vi "gauge_panel.vi"() -> ()   [LabVIEW 2017]
uses:
  slide_indicator.ctl
  <vilib>/Utility/miscctls.llb/LVPositionTypeDef.ctl
  global_variable_STOP.vi
  global_variable_GAUGE_PANEL_ERROR.vi
panel:
  out "TEMP_FILL_OX":T1 scale=-200.0..40.0
  out "TEMP_FILL_FU":T1 scale=-200.0..40.0
  out "Engine Temperatures (°C)":waveform(dbl)[](graph) caption="Waveform Chart"
  out "Engine Temperatures (°C)":waveform(dbl)[](graph) caption="Waveform Chart"
  out "Engine Pressures (PSI)":waveform(dbl)[](graph) caption="Waveform Chart"
  in  "PSI_ENGINE_8":dbl
  in  "PSI_ENGINE_7":dbl
  in  "PSI_ENGINE_6":dbl
  in  "PSI_ENGINE_5":dbl
  in  "PSI_ENGINE_4":dbl
  in  "PSI_ENGINE_3":dbl
  in  "PSI_ENGINE_2":dbl
  in  "PSI_ENGINE_1":dbl
  in  "TEMP_ENGINE_24":dbl
  in  "TEMP_ENGINE_23":dbl
  in  "TEMP_ENGINE_22":dbl
  in  "TEMP_ENGINE_21":dbl
  in  "TEMP_ENGINE_20":dbl
  in  "TEMP_ENGINE_19":dbl
  in  "TEMP_ENGINE_18":dbl
  in  "TEMP_ENGINE_17":dbl
  in  "TEMP_ENGINE_16":dbl
  in  "TEMP_ENGINE_15":dbl
  in  "TEMP_ENGINE_14":dbl
  in  "TEMP_ENGINE_13":dbl
  in  "TEMP_ENGINE_12":dbl
  in  "TEMP_ENGINE_11":dbl
  in  "TEMP_ENGINE_10":dbl
  in  "TEMP_ENGINE_9":dbl
  in  "TEMP_ENGINE_8":dbl
  in  "TEMP_ENGINE_7":dbl
  out "Calibration (LBF)":waveform(dbl)(graph) caption="Waveform Chart"
  out "Tank Pressures (PSI)":waveform(dbl)[](graph) caption="Waveform Chart"
  out "ACT_WINCH_DIR":bool
  out "ACT_WINCH_ON":bool
  out "LOAD_CALIBRATION":dbl
  out "ARMED":bool
  out "DAQ_ARM":bool
  out "TEMP_POSTCV_OX":T1 scale=-200.0..40.0
  out "TEMP_POSTCV_FU":T1 scale=-200.0..40.0
  out "TEMP_PRECV_OX":T1 scale=-200.0..40.0
  out "TEMP_PRECV_FU":T1 scale=-200.0..40.0
  out "LOAD_SUM":dbl
  out "TEMP_TANK_OX":T1 scale=-200.0..40.0
  out "TEMP_TANK_FU":T1 scale=-200.0..40.0
  out "PSI_KBOT_PURGE":T1 scale=0.0..3000.0
  out "PSI_KBOT_PRESS":T1 scale=0.0..3000.0
  out "PSI_REG_PNA":T1 scale=0.0..300.0
  out "PSI_KBOT_PNA":T1 scale=0.0..3000.0
  out "PSI_REG_PURGE":T1 scale=0.0..300.0
  out "PSI_POSTCV_OX":T1 scale=0.0..1500.0
  out "PSI_PRECV_OX":T1 scale=0.0..1500.0
  out "PSI_POSTCV_FU":T1 scale=0.0..1500.0
  out "PSI_PRECV_FU":T1 scale=0.0..1500.0
  out "PSI_TANK_OX":T1 scale=0.0..1500.0
  out "PSI_REG_OXPRESS":T1 scale=0.0..1500.0
  out "PSI_TANK_FU":T1 scale=0.0..1500.0
  out "PSI_REG_FUPRESS":T1 scale=0.0..1500.0
  out "Tank Temperatures (°C)":waveform(dbl)[](graph) caption="Waveform Chart"
  out "Thrust (LBF)":waveform(dbl)(graph) caption="Waveform Chart"
  # "DAQ ESTOP CONTROL"
  # "ESTOP HIT?"
  # "K-Bottle Pressures (PSI)"
  # "Post Regulator Pressures (PSI)"
  # "Fill Temperatures (°C)"
  # "Press"
  # "Purge"
  # "PNA"
  # "Purge"
  # "PNA"
  # "FU Press"
  # "OX Press"
  # "FU Fill"
  # "OX Fill"
  # "WINCH ON?"
  # "WINCH DIRECTION"
  # "Line Pressures (PSI)"
  # "Tank Pressures (PSI)"
  # "FU 1"
  # "FU 2"
  # "OX 1"
  # "OX 2"
  # "FU Tank"
  # "OX Tank"
  # "Line Temperatures (°C)"
  # "Tank Temperatures (°C)"
  # "FU 1"
  # "FU 2"
  # "OX 1"
  # "OX 2"
  # "FU Tank"
  # "OX Tank"
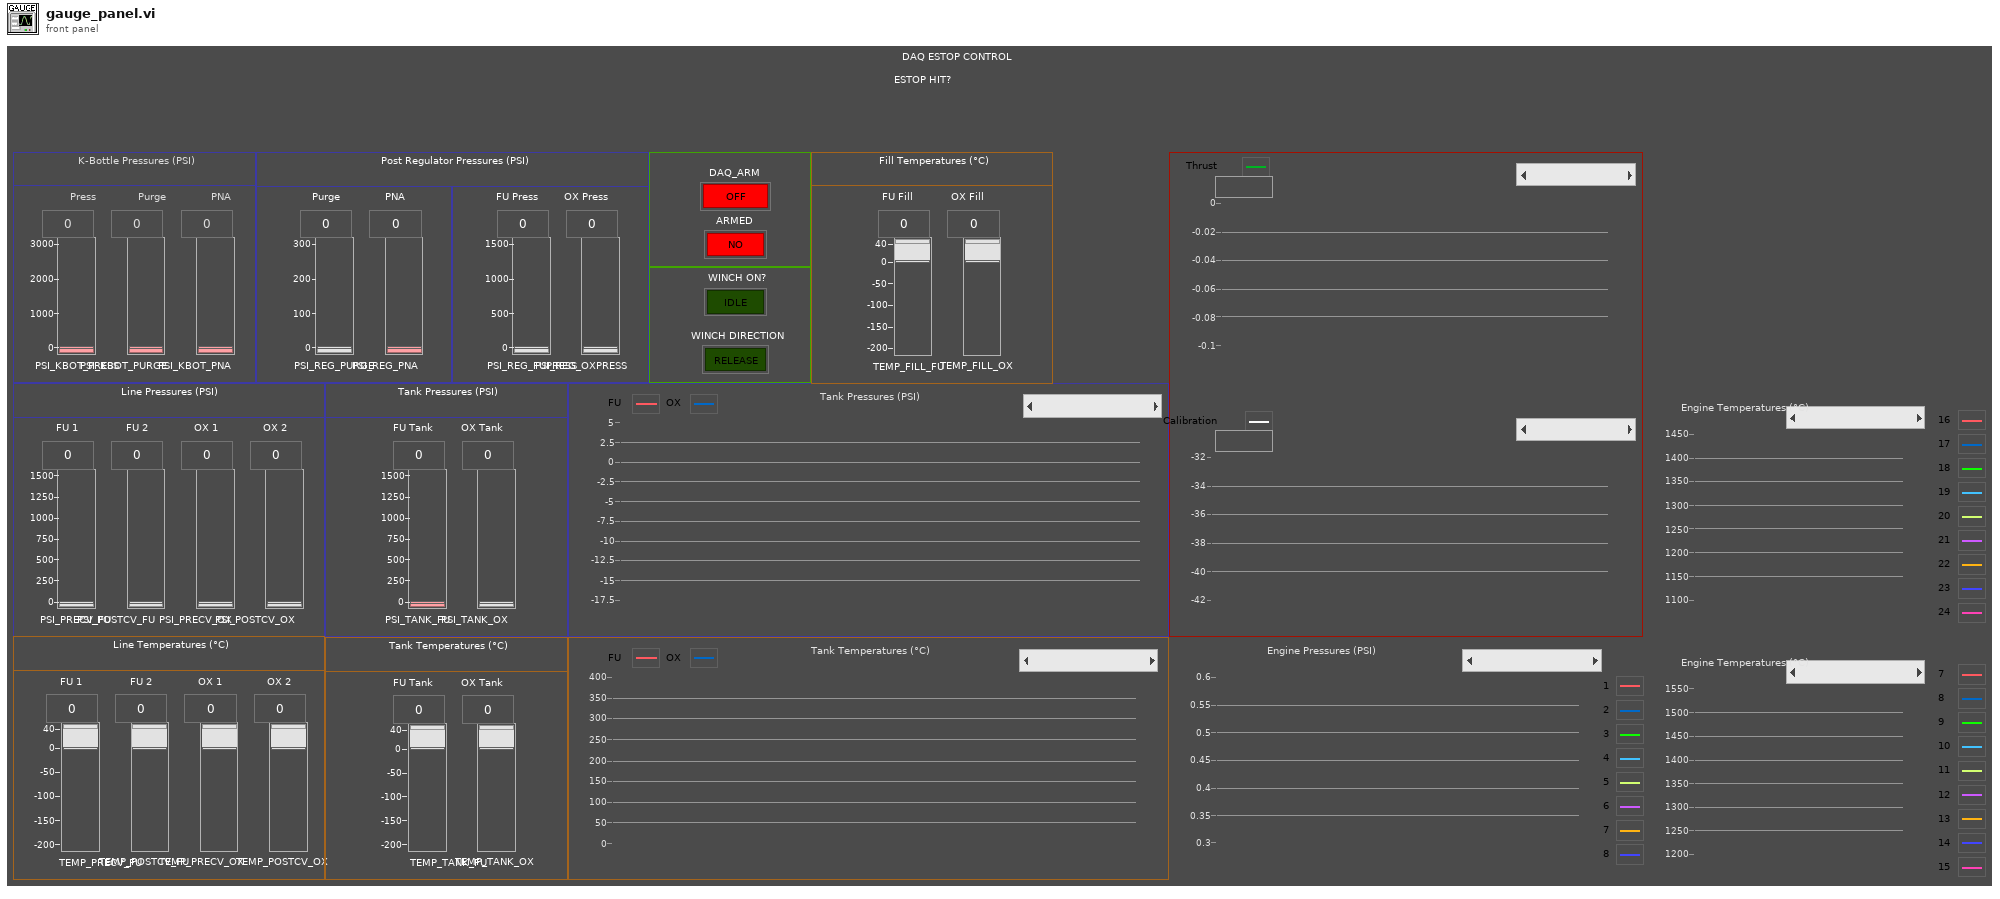
[diagram p1: front panel]
types:
  T1 = typedef "slide_indicator.ctl" = dbl
  T2 = typedef "LVPositionTypeDef.ctl" = cluster{"Left":i32, "Top":i32}
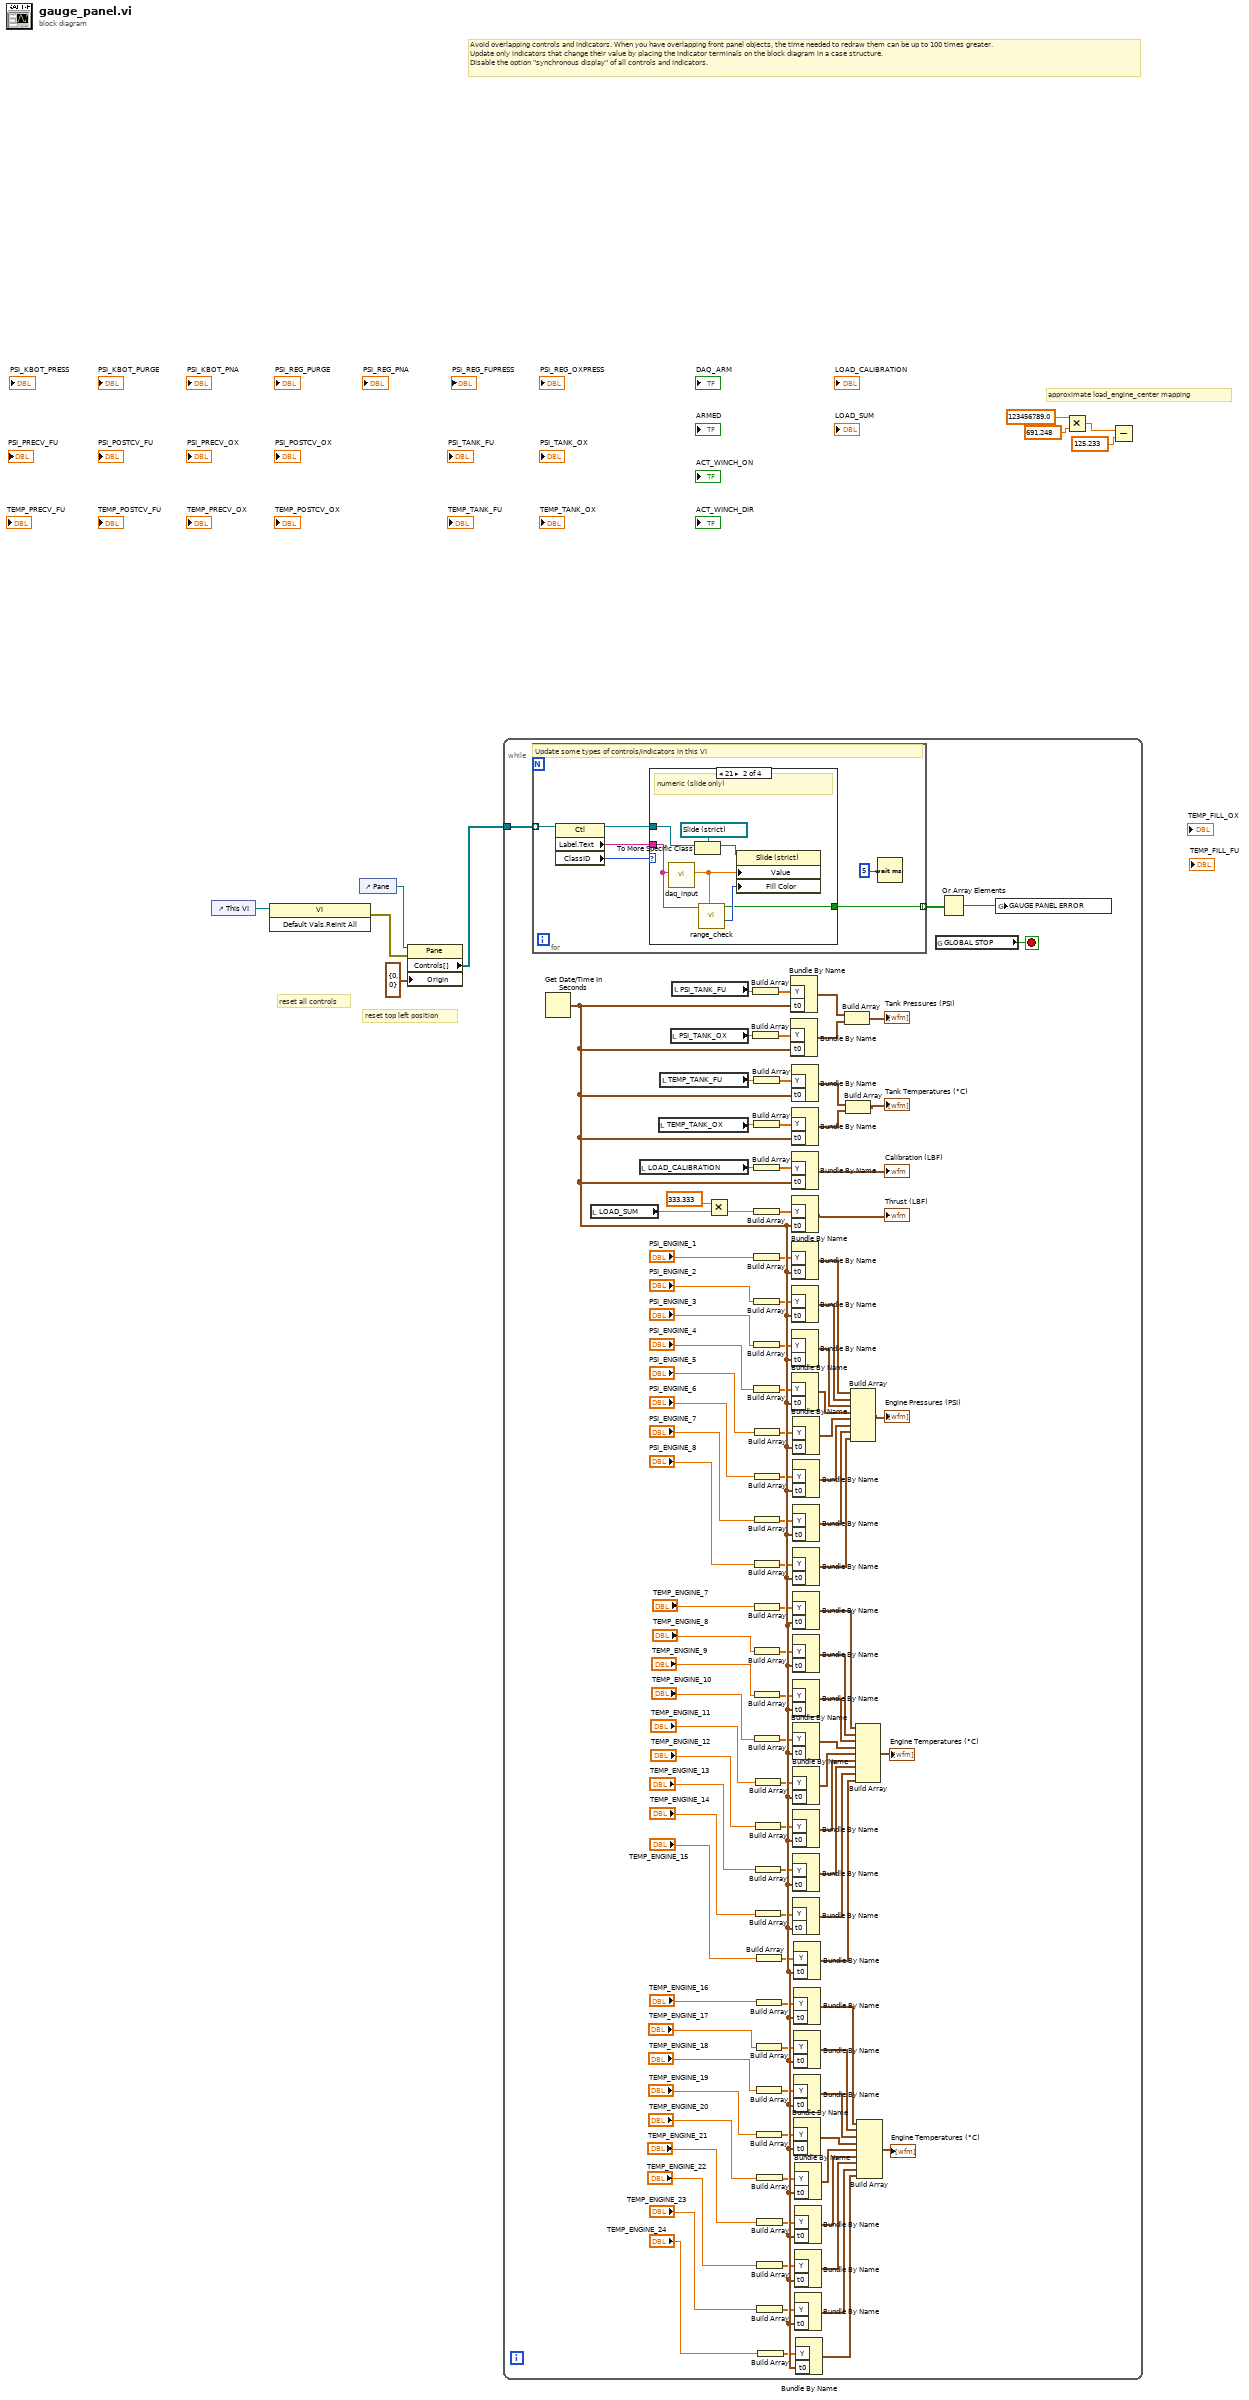
[diagram p0: block diagram]
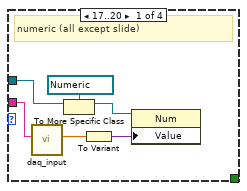
[diagram p2: hidden frame]
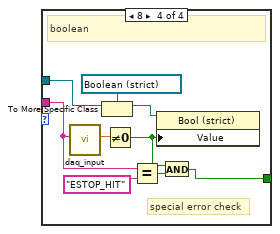
[diagram p4: hidden frame]
diagram:
  # "approximate load_engine_center mapping"
  # "reset top left position"
  # "reset all controls"
  # "Avoid overlapping controls and indicators. When you have overlapping front panel objects, the time needed to redraw them can be up to 100 times greater.\nUpdate only indicators that change their value by placing the indicator terminals on the block diagram in a case structure.\nDisable the option \"synchronous display\" of all controls and indicators."
  n1 = control-ref of="This VI"() -> (w7:refnum<vi>)
  n2 = invoke class="VI" method="Default Vals.Reinit All"(reference=w7) -> (error out=w9:errorcluster)  [unwired: 2 in, 2 out]
  n3 = control-ref of="Pane"() -> (w6:refnum<vi>)
  n4 = property class="Pane"(reference=w6, error in=w9, "Origin"=T2 {"Left"=0, "Top"=0} ("Position")) -> ("Controls[]"=w5:refnum<vi>[])  [unwired: 2 out]
  n5 = while {
    tunnel: w5 -> [w117]
    stop <- w116 stop-if-true
    n6 = for {
      tunnel: w117 -> [w121] mode=indexing
      tunnel: [w118] -> w115 mode=indexing
      # "Update some types of controls/indicators in this VI"
      n7 = property class="Ctl"(reference=w121) -> (reference out=w122:refnum<vi>, "Label.Text"=w123:string, "ClassID"=w119:u32)  [unwired: 1 in, 1 out]
      n8 = case shown="21" w119 {
        tunnel: w123 -> [w124 w133 _ w141]
        tunnel: w122 -> [w126 w134 _ w142]
        tunnel: [_ w130 _ w137] -> w118
        frame 17..20 {
          # "numeric (all except slide)"
          n9 = call "daq_input.vi"("channel"=w124) -> ("value"=w125:dbl)  [unwired: 9 in, 1 out]
          n10 = To More Specific Class(target class=refnum<vi> refnum ("Num Refnum"), reference=w126) -> (specific class reference=w129:refnum<vi>)  [unwired: 1 in, 1 out]
          n11 = To Variant(anything=w125) -> (Variant=w128:variant)
          n12 = property on="Property Node" class="Num"(reference=w129, "Value"=w128) -> ()  [unwired: 1 in, 2 out]
        }
        frame 21 {
          # "numeric (slide only)"
          n13 = call "daq_input.vi"("channel"=w133) -> ("value"=w132:dbl)  [unwired: 9 in, 1 out]
          n14 = To More Specific Class(target class=refnum<vi> refnum ("Slide Refnum"), reference=w134) -> (specific class reference=w136:refnum<vi>)  [unwired: 1 in, 1 out]
          n15 = call "range_check.vi"("data value"=w132, "config file key"=w133) -> ("color out"=w131:u32, "error?"=w130:bool)  [unwired: 8 in]
          n16 = property on="Property Node" class="Slide (strict)"(reference=w136, "Value"=w132, "Fill Color"=w131) -> ()  [unwired: 1 in, 2 out]
        }
        frame Default {
          # "do nothing"
          # "other"
        }
        frame 8 {
          # "special error check"
          # "boolean"
          n17 = call "daq_input.vi"("channel"=w141) -> ("value"=w145:dbl)  [unwired: 9 in, 1 out]
          n18 = To More Specific Class(target class=refnum<vi> refnum ("Bool Refnum"), reference=w142) -> (specific class reference=w143:refnum<vi>)  [unwired: 1 in, 1 out]
          n19 = Not Equal To 0?(x=w145) -> (x != 0?=w138:bool)
          n20 = Equal?(x=w141, y="ESTOP_HIT") -> (x = y?=w139:bool)
          n21 = property on="Property Node" class="Bool (strict)"(reference=w143, "Value"=w138) -> ()  [unwired: 1 in, 2 out]
          n22 = And(x=w138, y=w139) -> (x .and. y?=w137:bool)
        }
      }
      n23 = Wait (ms)(milliseconds to wait=u32 5) -> ()  [unwired: 1 out]
    }
    n24 = Get Date/Time In Seconds() -> (seconds since 1Jan1904=w111:timestamp)
    n25 = local read "LOAD_SUM"() -> (w12:dbl)
    n26 = local read "LOAD_CALIBRATION"() -> (w29:dbl)
    n27 = local read "TEMP_TANK_OX"() -> (w26:T1)
    n28 = local read "TEMP_TANK_FU"() -> (w25:T1)
    n29 = local read "PSI_TANK_OX"() -> (w18:T1)
    n30 = local read "PSI_TANK_FU"() -> (w17:T1)
    n31 = Multiply(x=333.333, y=w12) -> (x*y=w11:dbl)
    n32 = Build Array(w17) -> (w14:T1[])
    n33 = Build Array(w18) -> (w13:T1[])
    n34 = Build Array(w25) -> (w21:T1[])
    n35 = Build Array(w26) -> (w20:T1[])
    n36 = Build Array(w29) -> (w28:dbl[])
    n37 = Build Array(w11) -> (w27:dbl[])
    n38 = Build Array("PSI_ENGINE_1") -> (w33:dbl[])
    n39 = Build Array("PSI_ENGINE_2") -> (w32:dbl[])
    n40 = Build Array("PSI_ENGINE_3") -> (w37:dbl[])
    n41 = Build Array("PSI_ENGINE_4") -> (w36:dbl[])
    n42 = Build Array("PSI_ENGINE_5") -> (w43:dbl[])
    n43 = Build Array("PSI_ENGINE_6") -> (w42:dbl[])
    n44 = Build Array("PSI_ENGINE_7") -> (w45:dbl[])
    n45 = Build Array("PSI_ENGINE_8") -> (w44:dbl[])
    n46 = Build Array("TEMP_ENGINE_7") -> (w58:dbl[])
    n47 = Build Array("TEMP_ENGINE_8") -> (w57:dbl[])
    n48 = Build Array("TEMP_ENGINE_9") -> (w60:dbl[])
    n49 = Build Array("TEMP_ENGINE_10") -> (w59:dbl[])
    n50 = Build Array("TEMP_ENGINE_11") -> (w62:dbl[])
    n51 = Build Array("TEMP_ENGINE_12") -> (w61:dbl[])
    n52 = Build Array("TEMP_ENGINE_13") -> (w64:dbl[])
    n53 = Build Array("TEMP_ENGINE_14") -> (w63:dbl[])
    n54 = Build Array("TEMP_ENGINE_15") -> (w65:dbl[])
    n55 = Build Array("TEMP_ENGINE_16") -> (w76:dbl[])
    n56 = Build Array("TEMP_ENGINE_17") -> (w75:dbl[])
    n57 = Build Array("TEMP_ENGINE_18") -> (w78:dbl[])
    n58 = Build Array("TEMP_ENGINE_19") -> (w77:dbl[])
    n59 = Build Array("TEMP_ENGINE_20") -> (w80:dbl[])
    n60 = Build Array("TEMP_ENGINE_21") -> (w79:dbl[])
    n61 = Build Array("TEMP_ENGINE_22") -> (w82:dbl[])
    n62 = Build Array("TEMP_ENGINE_23") -> (w81:dbl[])
    n63 = Build Array("TEMP_ENGINE_24") -> (w83:dbl[])
    n64 = Bundle By Name("Y"=w14, "t0"=w111) -> (w16:waveform(dbl))  [unwired: 1 in]
    n65 = Bundle By Name("Y"=w13, "t0"=w111) -> (w15:waveform(dbl))  [unwired: 1 in]
    n66 = Bundle By Name("Y"=w21, "t0"=w111) -> (w23:waveform(dbl))  [unwired: 1 in]
    n67 = Bundle By Name("Y"=w20, "t0"=w111) -> (w22:waveform(dbl))  [unwired: 1 in]
    n68 = Bundle By Name("Y"=w28, "t0"=w111) -> (→"Calibration (LBF)":waveform(dbl))  [unwired: 1 in]
    n69 = Bundle By Name("Y"=w27, "t0"=w111) -> (→"Thrust (LBF)":waveform(dbl))  [unwired: 1 in]
    n70 = Bundle By Name("Y"=w33, "t0"=w111) -> (w35:waveform(dbl))  [unwired: 1 in]
    n71 = Bundle By Name("Y"=w32, "t0"=w111) -> (w34:waveform(dbl))  [unwired: 1 in]
    n72 = Bundle By Name("Y"=w37, "t0"=w111) -> (w55:waveform(dbl))  [unwired: 1 in]
    n73 = Bundle By Name("Y"=w36, "t0"=w111) -> (w54:waveform(dbl))  [unwired: 1 in]
    n74 = Bundle By Name("Y"=w43, "t0"=w111) -> (w53:waveform(dbl))  [unwired: 1 in]
    n75 = Bundle By Name("Y"=w42, "t0"=w111) -> (w52:waveform(dbl))  [unwired: 1 in]
    n76 = Bundle By Name("Y"=w45, "t0"=w111) -> (w51:waveform(dbl))  [unwired: 1 in]
    n77 = Bundle By Name("Y"=w44, "t0"=w111) -> (w50:waveform(dbl))  [unwired: 1 in]
    n78 = Bundle By Name("Y"=w58, "t0"=w111) -> (w66:waveform(dbl))  [unwired: 1 in]
    n79 = Bundle By Name("Y"=w57, "t0"=w111) -> (w67:waveform(dbl))  [unwired: 1 in]
    n80 = Bundle By Name("Y"=w60, "t0"=w111) -> (w68:waveform(dbl))  [unwired: 1 in]
    n81 = Bundle By Name("Y"=w59, "t0"=w111) -> (w69:waveform(dbl))  [unwired: 1 in]
    n82 = Bundle By Name("Y"=w62, "t0"=w111) -> (w70:waveform(dbl))  [unwired: 1 in]
    n83 = Bundle By Name("Y"=w61, "t0"=w111) -> (w71:waveform(dbl))  [unwired: 1 in]
    n84 = Bundle By Name("Y"=w64, "t0"=w111) -> (w72:waveform(dbl))  [unwired: 1 in]
    n85 = Bundle By Name("Y"=w63, "t0"=w111) -> (w73:waveform(dbl))  [unwired: 1 in]
    n86 = Bundle By Name("Y"=w65, "t0"=w111) -> (w74:waveform(dbl))  [unwired: 1 in]
    n87 = Bundle By Name("Y"=w76, "t0"=w111) -> (w84:waveform(dbl))  [unwired: 1 in]
    n88 = Bundle By Name("Y"=w75, "t0"=w111) -> (w85:waveform(dbl))  [unwired: 1 in]
    n89 = Bundle By Name("Y"=w78, "t0"=w111) -> (w86:waveform(dbl))  [unwired: 1 in]
    n90 = Bundle By Name("Y"=w77, "t0"=w111) -> (w87:waveform(dbl))  [unwired: 1 in]
    n91 = Bundle By Name("Y"=w80, "t0"=w111) -> (w88:waveform(dbl))  [unwired: 1 in]
    n92 = Bundle By Name("Y"=w79, "t0"=w111) -> (w89:waveform(dbl))  [unwired: 1 in]
    n93 = Bundle By Name("Y"=w82, "t0"=w111) -> (w90:waveform(dbl))  [unwired: 1 in]
    n94 = Bundle By Name("Y"=w81, "t0"=w111) -> (w91:waveform(dbl))  [unwired: 1 in]
    n95 = Bundle By Name("Y"=w83, "t0"=w111) -> (w92:waveform(dbl))  [unwired: 1 in]
    n96 = Build Array(w16, w15) -> (→"Tank Pressures (PSI)":waveform(dbl)[])
    n97 = Build Array(w23, w22) -> (→"Tank Temperatures (°C)":waveform(dbl)[])
    n98 = Build Array(w35, w34, w55, w54, w53, w52, w51, w50) -> (→"Engine Pressures (PSI)":waveform(dbl)[])
    n99 = Build Array(w66, w67, w68, w69, w70, w71, w72, w73, w74) -> (→"Engine Temperatures (°C)":waveform(dbl)[])
    n100 = Build Array(w84, w85, w86, w87, w88, w89, w90, w91, w92) -> (→"Engine Temperatures (°C)":waveform(dbl)[])
    n101 = global read "global_variable_STOP.vi" "GLOBAL STOP"() -> (w116:bool)
    n102 = Or Array Elements(Boolean array=w115) -> (logical OR=w114:bool)
    n103 = global write "global_variable_GAUGE_PANEL_ERROR.vi" "GAUGE PANEL ERROR"(w114) -> ()
  }
  n104 = Multiply(x=123456789.0, y=691.248) -> (x*y=w4:dbl)
  n105 = Subtract(x=w4, y=125.233) -> ()  [unwired: 1 out]
